vi "Process Array Elements - backup.vi"(5 "Read/Write Options":T1, 7 "Format String (%#0.15f)":string="%#0.15f", 8 "Error In":errorcluster, 9 "Name In":string, 10 "Array Variant":variant, 11 "Queue In":refnum<queue>) -> (0 "Error Out":errorcluster, 1 "Data Out":string, 3 "Queue Out":refnum<queue>)   [LabVIEW 2020]
doc: "This VI was created for use with the Read/Write Cluster VIs. It converts array elements of the cluster to strings to be written to file.\n\nFreeware from Moore Good Ideas, www.mooregoodideas.com. Do not remove this line."
uses:
  <vilib>/Utility/VariantDataType/VariantType.lvlib
  <vilib>/Utility/Data Type/NI_Data Type.lvlib
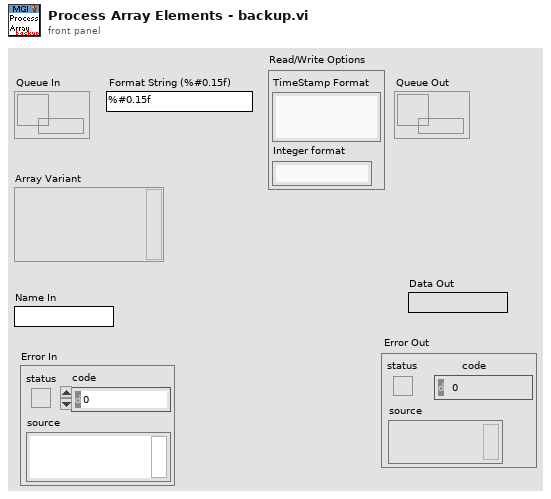
[diagram p1: front panel]
types:
  T1 = cluster{"TimeStamp Format":string, "Integer format":string}
  T2 = typedef "NI_Data Type.lvlib/Data Type.ctl" = enum8{"Invalid Type", "Void", "I8", "I16", "I32", "I64", "U8", "U16", "U32", "U64", "Single Float", "Double Float", "Extended Float", "Single Complex", "Double Complex", "Extended Complex", "Enum U8", "Enum U16", "Enum U32", "Enum U64", "Single Float With Unit", "Double Float With Unit", "Extended Float With Unit", "Single Complex with Unit", "Double Complex with Unit", "Extended Complex with Unit", "Boolean", "String", "Path", "Picture", "Tag", "Array", "Cluster", "Variant", "LV Variant", "Waveform", "Timestamp", "Digital Waveform", "Digital Data", "ExpressData", "Refnum", "External Data", "VI", "Poly VI", "LabVIEW Class Instance", "Fixed Point", "Set Collection", "Map Collection"}
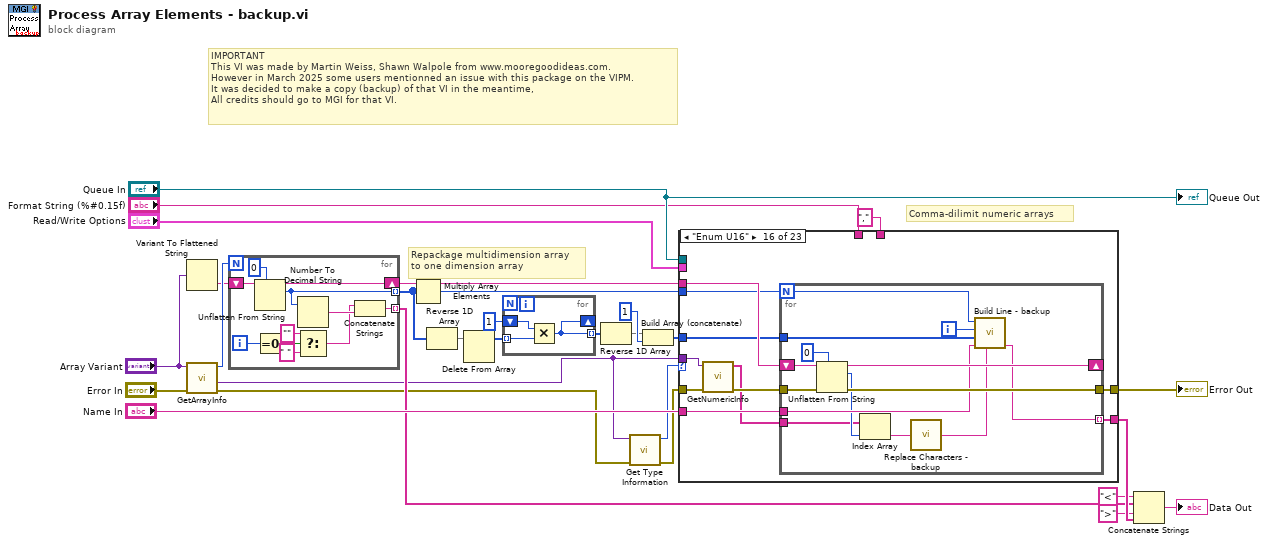
[diagram p0: block diagram]
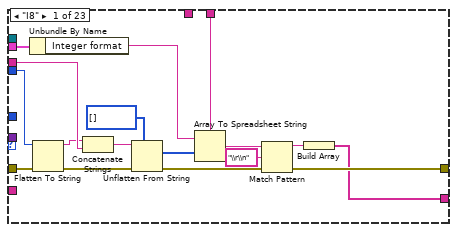
[diagram p2: hidden frame]
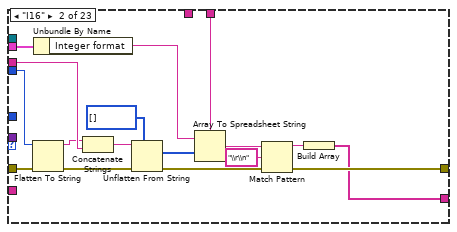
[diagram p3: hidden frame]
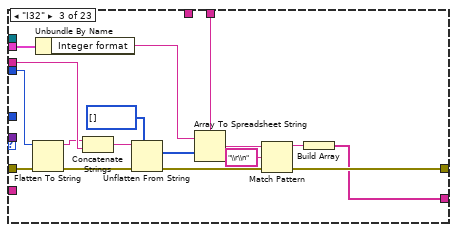
[diagram p4: hidden frame]
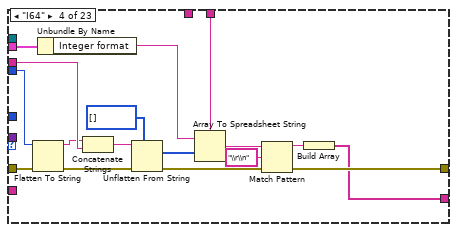
[diagram p5: hidden frame]
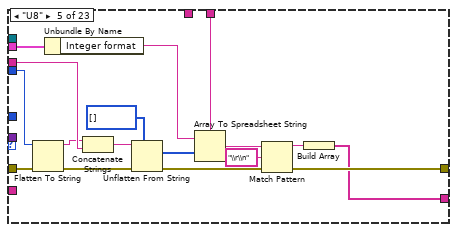
[diagram p6: hidden frame]
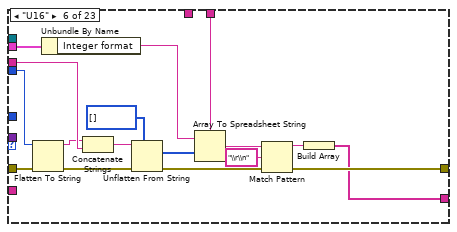
[diagram p7: hidden frame]
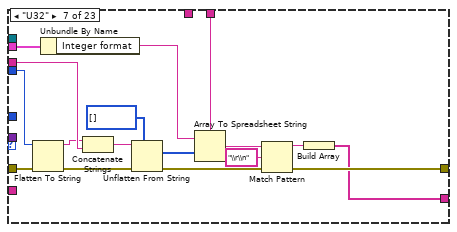
[diagram p8: hidden frame]
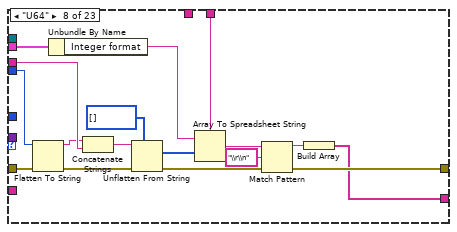
[diagram p9: hidden frame]
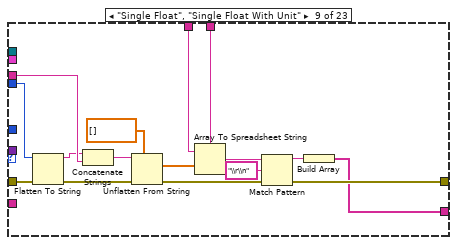
[diagram p10: hidden frame]
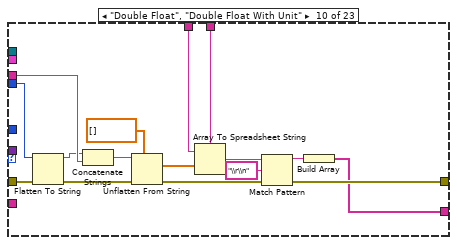
[diagram p11: hidden frame]
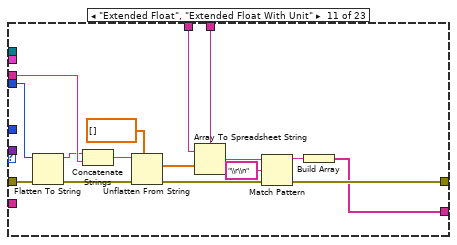
[diagram p12: hidden frame]
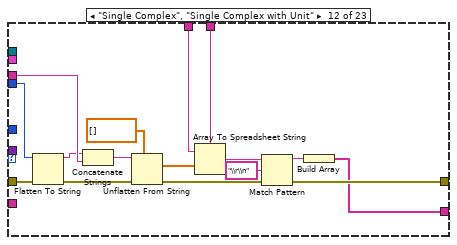
[diagram p13: hidden frame]
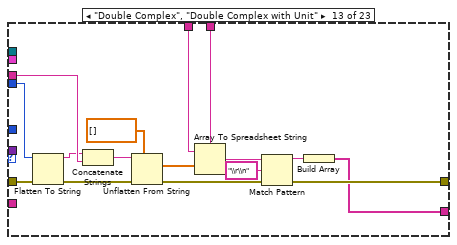
[diagram p14: hidden frame]
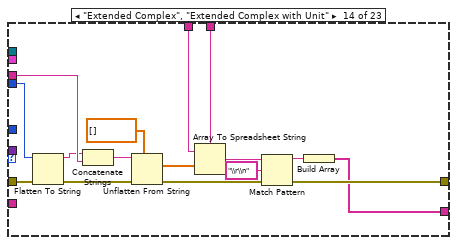
[diagram p15: hidden frame]
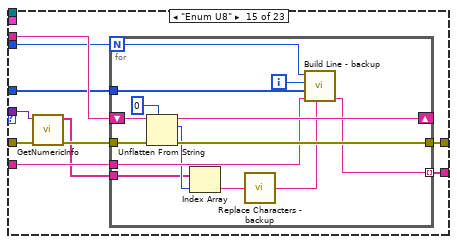
[diagram p16: hidden frame]
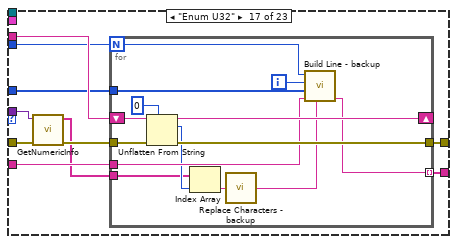
[diagram p17: hidden frame]
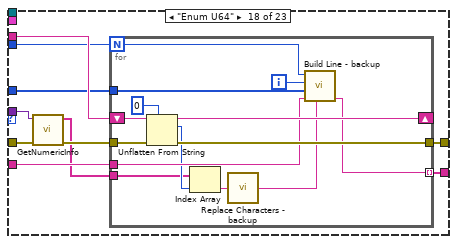
[diagram p18: hidden frame]
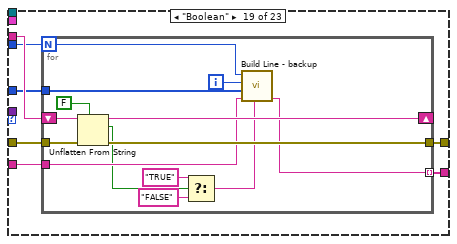
[diagram p19: hidden frame]
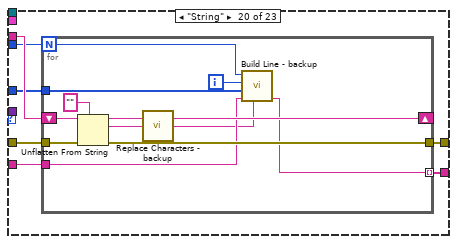
[diagram p20: hidden frame]
diagram:
  # "IMPORTANT\nThis VI was made by Martin Weiss, Shawn Walpole from www.mooregoodideas.com.\nHowever in March 2025 some users mentionned an issue with this package on the VIPM.\nIt was decided to make a copy (backup) of that VI in the meantime,\nAll credits should go to MGI for that VI."
  # "Comma-dilimit numeric arrays"
  # "Repackage multidimension array\nto one dimension array"
  n1 = Variant To Flattened String(Variant="Array Variant") -> (data string=w26:string)  [unwired: 1 out]
  n2 = call <vilib>:"GetArrayInfo.vi"("error in (no error)"="Error In", "Variant"="Array Variant") -> ("error out"=w3:errorcluster, "ArrayElement"=w4:variant, "NDims"=w27:i32)  [unwired: 6 in, 1 out]
  n3 = for {
    N: w27 -> [_]
    shift-right: [w38] -> w25
    shift-left: w26 -> [w39]
    tunnel: [w35] -> w14 mode=indexing
    tunnel: [w36] -> w10 mode=indexing
    i -> [w34]
    n4 = Unflatten From String(type=u32 0, binary string=w39) -> (rest of the binary string=w38:string, value=w35:u32)  [unwired: 3 in, 1 out]
    n5 = Equal To 0?(x=w34) -> (x = 0?=w33:bool)
    n6 = Number To Decimal String(number=w35) -> (decimal integer string=w37:string)  [unwired: 1 in]
    n7 = Select(t="", s=w33, f=" ") -> (s? t:f=w31:string)
    n8 = Concatenate Strings(w31, w37) -> (w36:string)
  }
  n9 = Multiply Array Elements(1:w14) -> (0:w24:u32)
  n10 = Reverse 1D Array(array=w14) -> (reversed array=w15:u32[])
  n11 = Delete From Array(array=w15) -> (array with subset deleted=w16:u32[])  [unwired: 2 in, 1 out]
  n12 = for {
    tunnel: w16 -> [w43] mode=indexing
    shift-right: [w41] -> _
    shift-left: i8 1 -> [w42]
    tunnel: [w41] -> w18 mode=indexing
    n13 = Multiply(x=w42, y=w43) -> (x*y=w41:u32)
  }
  n14 = Reverse 1D Array(array=w18) -> (reversed array=w19:u32[])
  n15 = call <vilib>:"Get Type Information.vi"("error in (no error)"=w3, "variant"=w4) -> ("error out"=w1:errorcluster, "type"=w2:T2)  [unwired: 5 in, 3 out]
  n16 = Build Array (concatenate)(w19, i8 1) -> (w13:u32[])
  n17 = case shown="\"Enum U16\"" w2 {
    tunnel: [w59 w75 w91 w107 w123 w139 w155 w171 w186 w201 w216 w231 w246 w261 w271 w295 w319 w343 w364 w385 w404 w420 w430] -> w12
    tunnel: w1 -> [w48 w64 w80 w96 w112 w128 w144 w160 w175 w190 w205 w220 w235 w250 w264 w288 w312 w336 w363 w384 w403 w420 w438]
    tunnel: w25 -> [w58 w74 w90 w106 w122 w138 w154 w170 w185 w200 w215 w230 w245 w260 w270 w294 w318 w342 w362 w383 w402 w419 w425]
    tunnel: w24 -> [w57 w73 w89 w105 w121 w137 w153 w169 w184 w199 w214 w229 w244 w259 w269 w293 w317 w341 w361 w382 w401 _ w437]
    tunnel: "Name In" -> [_ _ _ _ _ _ _ _ _ _ _ _ _ _ w268 w292 w316 w340 w360 w381 w400 _ w436]
    tunnel: [w56 w72 w88 w104 w120 w136 w152 w168 w183 w198 w213 w228 w243 w258 w266 w290 w314 w338 w358 w379 w398 w418 _] -> w22
    tunnel: w13 -> [_ _ _ _ _ _ _ _ _ _ _ _ _ _ w267 w291 w315 w339 w359 w380 w399 _ w435]
    tunnel: "Queue In" -> [_ _ _ _ _ _ _ _ _ _ _ _ _ _ _ _ _ _ _ _ _ _ w431]
    tunnel: w4 -> [_ _ _ _ _ _ _ _ _ _ _ _ _ _ w265 w289 w313 w337 _ _ _ _ w428]
    tunnel: "Format String (%#0.15f)" -> [_ _ _ _ _ _ _ _ w173 w188 w203 w218 w233 w248 _ _ _ _ _ _ _ _ _]
    tunnel: "," ("delimiter (Tab)") -> [w46 w62 w78 w94 w110 w126 w142 w158 w172 w187 w202 w217 w232 w247 _ _ _ _ _ _ _ _ _]
    tunnel: "Read/Write Options" -> [w45 w61 w77 w93 w109 w125 w141 w157 _ _ _ _ _ _ _ _ _ _ _ _ _ _ _]
    frame "I8" {
      n18 = Unbundle By Name(w45) -> ("Integer format"=w44:string)
      n19 = Flatten To String(anything=w57, error in (no error)=w48) -> (data string=w53:string, error out=w47:errorcluster)  [unwired: 2 in, 1 out]
      n20 = Concatenate Strings(w53, w58) -> (w54:string)
      n21 = Unflatten From String(type=i8[] [], binary string=w54, error in (no error)=w47) -> (value=w50:i8[], error out=w59:errorcluster)  [unwired: 2 in, 1 out]
      n22 = Array To Spreadsheet String(delimiter (Tab)=w46, array=w50, 3:w44) -> (spreadsheet string=w52:string)
      n23 = Match Pattern(string=w52, regular expression="\\r\\n") -> (before substring=w49:string)  [unwired: 1 in, 3 out]
      n24 = Build Array(w49) -> (w56:string[])
    }
    frame "I16" {
      n25 = Flatten To String(anything=w73, error in (no error)=w64) -> (data string=w69:string, error out=w63:errorcluster)  [unwired: 2 in, 1 out]
      n26 = Unbundle By Name(w61) -> ("Integer format"=w60:string)
      n27 = Concatenate Strings(w69, w74) -> (w70:string)
      n28 = Unflatten From String(type=i16[] [], binary string=w70, error in (no error)=w63) -> (value=w66:i16[], error out=w75:errorcluster)  [unwired: 2 in, 1 out]
      n29 = Array To Spreadsheet String(delimiter (Tab)=w62, array=w66, 3:w60) -> (spreadsheet string=w68:string)
      n30 = Match Pattern(string=w68, regular expression="\\r\\n") -> (before substring=w65:string)  [unwired: 1 in, 3 out]
      n31 = Build Array(w65) -> (w72:string[])
    }
    frame "I32" {
      n32 = Flatten To String(anything=w89, error in (no error)=w80) -> (data string=w85:string, error out=w79:errorcluster)  [unwired: 2 in, 1 out]
      n33 = Unbundle By Name(w77) -> ("Integer format"=w76:string)
      n34 = Concatenate Strings(w85, w90) -> (w86:string)
      n35 = Unflatten From String(type=i32[] [], binary string=w86, error in (no error)=w79) -> (value=w82:i32[], error out=w91:errorcluster)  [unwired: 2 in, 1 out]
      n36 = Array To Spreadsheet String(delimiter (Tab)=w78, array=w82, 3:w76) -> (spreadsheet string=w84:string)
      n37 = Match Pattern(string=w84, regular expression="\\r\\n") -> (before substring=w81:string)  [unwired: 1 in, 3 out]
      n38 = Build Array(w81) -> (w88:string[])
    }
    frame "I64" {
      n39 = Flatten To String(anything=w105, error in (no error)=w96) -> (data string=w101:string, error out=w95:errorcluster)  [unwired: 2 in, 1 out]
      n40 = Unbundle By Name(w93) -> ("Integer format"=w92:string)
      n41 = Concatenate Strings(w101, w106) -> (w102:string)
      n42 = Unflatten From String(type=i64[] [], binary string=w102, error in (no error)=w95) -> (value=w98:i64[], error out=w107:errorcluster)  [unwired: 2 in, 1 out]
      n43 = Array To Spreadsheet String(delimiter (Tab)=w94, array=w98, 3:w92) -> (spreadsheet string=w100:string)
      n44 = Match Pattern(string=w100, regular expression="\\r\\n") -> (before substring=w97:string)  [unwired: 1 in, 3 out]
      n45 = Build Array(w97) -> (w104:string[])
    }
    frame "U8" {
      n46 = Flatten To String(anything=w121, error in (no error)=w112) -> (data string=w117:string, error out=w111:errorcluster)  [unwired: 2 in, 1 out]
      n47 = Unbundle By Name(w109) -> ("Integer format"=w108:string)
      n48 = Concatenate Strings(w117, w122) -> (w118:string)
      n49 = Unflatten From String(type=u8[] [], binary string=w118, error in (no error)=w111) -> (value=w114:u8[], error out=w123:errorcluster)  [unwired: 2 in, 1 out]
      n50 = Array To Spreadsheet String(delimiter (Tab)=w110, array=w114, 3:w108) -> (spreadsheet string=w116:string)
      n51 = Match Pattern(string=w116, regular expression="\\r\\n") -> (before substring=w113:string)  [unwired: 1 in, 3 out]
      n52 = Build Array(w113) -> (w120:string[])
    }
    frame "U16" {
      n53 = Flatten To String(anything=w137, error in (no error)=w128) -> (data string=w133:string, error out=w127:errorcluster)  [unwired: 2 in, 1 out]
      n54 = Unbundle By Name(w125) -> ("Integer format"=w124:string)
      n55 = Concatenate Strings(w133, w138) -> (w134:string)
      n56 = Unflatten From String(type=u16[] [], binary string=w134, error in (no error)=w127) -> (value=w130:u16[], error out=w139:errorcluster)  [unwired: 2 in, 1 out]
      n57 = Array To Spreadsheet String(delimiter (Tab)=w126, array=w130, 3:w124) -> (spreadsheet string=w132:string)
      n58 = Match Pattern(string=w132, regular expression="\\r\\n") -> (before substring=w129:string)  [unwired: 1 in, 3 out]
      n59 = Build Array(w129) -> (w136:string[])
    }
    frame "U32" {
      n60 = Flatten To String(anything=w153, error in (no error)=w144) -> (data string=w149:string, error out=w143:errorcluster)  [unwired: 2 in, 1 out]
      n61 = Unbundle By Name(w141) -> ("Integer format"=w140:string)
      n62 = Concatenate Strings(w149, w154) -> (w150:string)
      n63 = Unflatten From String(type=u32[] [], binary string=w150, error in (no error)=w143) -> (value=w146:u32[], error out=w155:errorcluster)  [unwired: 2 in, 1 out]
      n64 = Array To Spreadsheet String(delimiter (Tab)=w142, array=w146, 3:w140) -> (spreadsheet string=w148:string)
      n65 = Match Pattern(string=w148, regular expression="\\r\\n") -> (before substring=w145:string)  [unwired: 1 in, 3 out]
      n66 = Build Array(w145) -> (w152:string[])
    }
    frame "U64" {
      n67 = Flatten To String(anything=w169, error in (no error)=w160) -> (data string=w165:string, error out=w159:errorcluster)  [unwired: 2 in, 1 out]
      n68 = Unbundle By Name(w157) -> ("Integer format"=w156:string)
      n69 = Concatenate Strings(w165, w170) -> (w166:string)
      n70 = Unflatten From String(type=u64[] [], binary string=w166, error in (no error)=w159) -> (value=w162:u64[], error out=w171:errorcluster)  [unwired: 2 in, 1 out]
      n71 = Array To Spreadsheet String(delimiter (Tab)=w158, array=w162, 3:w156) -> (spreadsheet string=w164:string)
      n72 = Match Pattern(string=w164, regular expression="\\r\\n") -> (before substring=w161:string)  [unwired: 1 in, 3 out]
      n73 = Build Array(w161) -> (w168:string[])
    }
    frame "Single Float", "Single Float With Unit" {
      n74 = Flatten To String(anything=w184, error in (no error)=w175) -> (data string=w180:string, error out=w174:errorcluster)  [unwired: 2 in, 1 out]
      n75 = Concatenate Strings(w180, w185) -> (w181:string)
      n76 = Unflatten From String(type=sgl[] [], binary string=w181, error in (no error)=w174) -> (value=w177:sgl[], error out=w186:errorcluster)  [unwired: 2 in, 1 out]
      n77 = Array To Spreadsheet String(delimiter (Tab)=w172, array=w177, 3:w173) -> (spreadsheet string=w179:string)
      n78 = Match Pattern(string=w179, regular expression="\\r\\n") -> (before substring=w176:string)  [unwired: 1 in, 3 out]
      n79 = Build Array(w176) -> (w183:string[])
    }
    frame "Double Float", "Double Float With Unit" {
      n80 = Flatten To String(anything=w199, error in (no error)=w190) -> (data string=w195:string, error out=w189:errorcluster)  [unwired: 2 in, 1 out]
      n81 = Concatenate Strings(w195, w200) -> (w196:string)
      n82 = Unflatten From String(type=dbl[] [], binary string=w196, error in (no error)=w189) -> (value=w192:dbl[], error out=w201:errorcluster)  [unwired: 2 in, 1 out]
      n83 = Array To Spreadsheet String(delimiter (Tab)=w187, array=w192, 3:w188) -> (spreadsheet string=w194:string)
      n84 = Match Pattern(string=w194, regular expression="\\r\\n") -> (before substring=w191:string)  [unwired: 1 in, 3 out]
      n85 = Build Array(w191) -> (w198:string[])
    }
    frame "Extended Float", "Extended Float With Unit" {
      n86 = Flatten To String(anything=w214, error in (no error)=w205) -> (data string=w210:string, error out=w204:errorcluster)  [unwired: 2 in, 1 out]
      n87 = Concatenate Strings(w210, w215) -> (w211:string)
      n88 = Unflatten From String(type=ext[] [], binary string=w211, error in (no error)=w204) -> (value=w207:ext[], error out=w216:errorcluster)  [unwired: 2 in, 1 out]
      n89 = Array To Spreadsheet String(delimiter (Tab)=w202, array=w207, 3:w203) -> (spreadsheet string=w209:string)
      n90 = Match Pattern(string=w209, regular expression="\\r\\n") -> (before substring=w206:string)  [unwired: 1 in, 3 out]
      n91 = Build Array(w206) -> (w213:string[])
    }
    frame "Single Complex", "Single Complex with Unit" {
      n92 = Flatten To String(anything=w229, error in (no error)=w220) -> (data string=w225:string, error out=w219:errorcluster)  [unwired: 2 in, 1 out]
      n93 = Concatenate Strings(w225, w230) -> (w226:string)
      n94 = Unflatten From String(type=csg[] [], binary string=w226, error in (no error)=w219) -> (value=w222:csg[], error out=w231:errorcluster)  [unwired: 2 in, 1 out]
      n95 = Array To Spreadsheet String(delimiter (Tab)=w217, array=w222, 3:w218) -> (spreadsheet string=w224:string)
      n96 = Match Pattern(string=w224, regular expression="\\r\\n") -> (before substring=w221:string)  [unwired: 1 in, 3 out]
      n97 = Build Array(w221) -> (w228:string[])
    }
    frame "Double Complex", "Double Complex with Unit" {
      n98 = Flatten To String(anything=w244, error in (no error)=w235) -> (data string=w240:string, error out=w234:errorcluster)  [unwired: 2 in, 1 out]
      n99 = Concatenate Strings(w240, w245) -> (w241:string)
      n100 = Unflatten From String(type=cdb[] [], binary string=w241, error in (no error)=w234) -> (value=w237:cdb[], error out=w246:errorcluster)  [unwired: 2 in, 1 out]
      n101 = Array To Spreadsheet String(delimiter (Tab)=w232, array=w237, 3:w233) -> (spreadsheet string=w239:string)
      n102 = Match Pattern(string=w239, regular expression="\\r\\n") -> (before substring=w236:string)  [unwired: 1 in, 3 out]
      n103 = Build Array(w236) -> (w243:string[])
    }
    frame "Extended Complex", "Extended Complex with Unit" {
      n104 = Flatten To String(anything=w259, error in (no error)=w250) -> (data string=w255:string, error out=w249:errorcluster)  [unwired: 2 in, 1 out]
      n105 = Concatenate Strings(w255, w260) -> (w256:string)
      n106 = Unflatten From String(type=cxt[] [], binary string=w256, error in (no error)=w249) -> (value=w252:cxt[], error out=w261:errorcluster)  [unwired: 2 in, 1 out]
      n107 = Array To Spreadsheet String(delimiter (Tab)=w247, array=w252, 3:w248) -> (spreadsheet string=w254:string)
      n108 = Match Pattern(string=w254, regular expression="\\r\\n") -> (before substring=w251:string)  [unwired: 1 in, 3 out]
      n109 = Build Array(w251) -> (w258:string[])
    }
    frame "Enum U8" {
      n110 = call <vilib>:"GetNumericInfo.vi"("error in (no error)"=w264, "Variant"=w265) -> ("error out"=w263:errorcluster, "EnumNames"=w262:string[])  [unwired: 6 in, 2 out]
      n111 = for {
        N: w269 -> [w281]
        tunnel: [w282] -> w271
        tunnel: w263 -> [w283]
        shift-right: [w284] -> _
        shift-left: w270 -> [w285]
        tunnel: w268 -> [w277]
        tunnel: [w278] -> w266 mode=indexing
        tunnel: w267 -> [w279]
        tunnel: w262 -> [w274]
        i -> [w280]
        n112 = Unflatten From String(type=u8 0, binary string=w285, error in (no error)=w283) -> (rest of the binary string=w284:string, value=w275:u8, error out=w282:errorcluster)  [unwired: 2 in]
        n113 = Index Array(array=w274, index=w275) -> (element=w273:string)
        n114 = call "Replace Characters - backup.vi"("String In"=w273) -> ("String Out"=w272:string)  [unwired: 1 in]
        n115 = call "Build Line - backup.vi"("Value String (\"\")"=w272, "Name In"=w277, "Array"=w279, "Iteration"=w280, "Iterations"=w281) -> ("Line"=w278:string)  [unwired: 5 in, 1 out]
      }
    }
    frame "Enum U16" {
      n116 = call <vilib>:"GetNumericInfo.vi"("error in (no error)"=w288, "Variant"=w289) -> ("error out"=w287:errorcluster, "EnumNames"=w286:string[])  [unwired: 6 in, 2 out]
      n117 = for {
        N: w293 -> [w305]
        tunnel: [w306] -> w295
        tunnel: w287 -> [w307]
        shift-right: [w308] -> _
        shift-left: w294 -> [w309]
        tunnel: w292 -> [w301]
        tunnel: [w302] -> w290 mode=indexing
        tunnel: w291 -> [w303]
        tunnel: w286 -> [w298]
        i -> [w304]
        n118 = Unflatten From String(type=u16 0, binary string=w309, error in (no error)=w307) -> (rest of the binary string=w308:string, value=w299:u16, error out=w306:errorcluster)  [unwired: 2 in]
        n119 = Index Array(array=w298, index=w299) -> (element=w297:string)
        n120 = call "Replace Characters - backup.vi"("String In"=w297) -> ("String Out"=w296:string)  [unwired: 1 in]
        n121 = call "Build Line - backup.vi"("Value String (\"\")"=w296, "Name In"=w301, "Array"=w303, "Iteration"=w304, "Iterations"=w305) -> ("Line"=w302:string)  [unwired: 5 in, 1 out]
      }
    }
    frame "Enum U32" {
      n122 = call <vilib>:"GetNumericInfo.vi"("error in (no error)"=w312, "Variant"=w313) -> ("error out"=w311:errorcluster, "EnumNames"=w310:string[])  [unwired: 6 in, 2 out]
      n123 = for {
        N: w317 -> [w329]
        tunnel: [w330] -> w319
        tunnel: w311 -> [w331]
        shift-right: [w332] -> _
        shift-left: w318 -> [w333]
        tunnel: w316 -> [w325]
        tunnel: [w326] -> w314 mode=indexing
        tunnel: w315 -> [w327]
        tunnel: w310 -> [w322]
        i -> [w328]
        n124 = Unflatten From String(type=u32 0, binary string=w333, error in (no error)=w331) -> (rest of the binary string=w332:string, value=w323:u32, error out=w330:errorcluster)  [unwired: 2 in]
        n125 = Index Array(array=w322, index=w323) -> (element=w321:string)
        n126 = call "Replace Characters - backup.vi"("String In"=w321) -> ("String Out"=w320:string)  [unwired: 1 in]
        n127 = call "Build Line - backup.vi"("Value String (\"\")"=w320, "Name In"=w325, "Array"=w327, "Iteration"=w328, "Iterations"=w329) -> ("Line"=w326:string)  [unwired: 5 in, 1 out]
      }
    }
    frame "Enum U64" {
      n128 = call <vilib>:"GetNumericInfo.vi"("error in (no error)"=w336, "Variant"=w337) -> ("error out"=w335:errorcluster, "EnumNames"=w334:string[])  [unwired: 6 in, 2 out]
      n129 = for {
        N: w341 -> [w353]
        tunnel: [w354] -> w343
        tunnel: w335 -> [w355]
        shift-right: [w356] -> _
        shift-left: w342 -> [w357]
        tunnel: w340 -> [w349]
        tunnel: [w350] -> w338 mode=indexing
        tunnel: w339 -> [w351]
        tunnel: w334 -> [w346]
        i -> [w352]
        n130 = Unflatten From String(type=u64 0, binary string=w357, error in (no error)=w355) -> (rest of the binary string=w356:string, value=w347:u64, error out=w354:errorcluster)  [unwired: 2 in]
        n131 = Index Array(array=w346, index=w347) -> (element=w345:string)
        n132 = call "Replace Characters - backup.vi"("String In"=w345) -> ("String Out"=w344:string)  [unwired: 1 in]
        n133 = call "Build Line - backup.vi"("Value String (\"\")"=w344, "Name In"=w349, "Array"=w351, "Iteration"=w352, "Iterations"=w353) -> ("Line"=w350:string)  [unwired: 5 in, 1 out]
      }
    }
    frame "Boolean" {
      n134 = for {
        N: w361 -> [w374]
        tunnel: [w375] -> w364
        tunnel: w363 -> [w376]
        shift-right: [w377] -> _
        shift-left: w362 -> [w378]
        tunnel: w360 -> [w370]
        tunnel: [w371] -> w358 mode=indexing
        tunnel: w359 -> [w372]
        i -> [w373]
        n135 = Unflatten From String(type=FALSE, binary string=w378, error in (no error)=w376) -> (rest of the binary string=w377:string, value=w366:bool, error out=w375:errorcluster)  [unwired: 2 in]
        n136 = Select(t="TRUE", s=w366, f="FALSE") -> (s? t:f=w365:string)
        n137 = call "Build Line - backup.vi"("Value String (\"\")"=w365, "Name In"=w370, "Array"=w372, "Iteration"=w373, "Iterations"=w374) -> ("Line"=w371:string)  [unwired: 5 in, 1 out]
      }
    }
    frame "String" {
      n138 = for {
        N: w382 -> [w393]
        tunnel: [w394] -> w385
        tunnel: w384 -> [w395]
        shift-right: [w396] -> _
        shift-left: w383 -> [w397]
        tunnel: w381 -> [w389]
        tunnel: [w390] -> w379 mode=indexing
        tunnel: w380 -> [w391]
        i -> [w392]
        n139 = Unflatten From String(type="", binary string=w397, error in (no error)=w395) -> (rest of the binary string=w396:string, value=w387:string, error out=w394:errorcluster)  [unwired: 2 in]
        n140 = call "Replace Characters - backup.vi"("String In"=w387) -> ("String Out"=w386:string)  [unwired: 1 in]
        n141 = call "Build Line - backup.vi"("Value String (\"\")"=w386, "Name In"=w389, "Array"=w391, "Iteration"=w392, "Iterations"=w393) -> ("Line"=w390:string)  [unwired: 5 in, 1 out]
      }
    }
    frame "Path" {
      n142 = for {
        N: w401 -> [w413]
        tunnel: [w414] -> w404
        tunnel: w403 -> [w415]
        shift-right: [w416] -> _
        shift-left: w402 -> [w417]
        tunnel: w400 -> [w409]
        tunnel: [w410] -> w398 mode=indexing
        tunnel: w399 -> [w411]
        i -> [w412]
        n143 = Unflatten From String(type=path "", binary string=w417, error in (no error)=w415) -> (rest of the binary string=w416:string, value=w407:path, error out=w414:errorcluster)  [unwired: 2 in]
        n144 = Path To String(path=w407) -> (string=w406:string)
        n145 = call "Replace Characters - backup.vi"("String In"=w406) -> ("String Out"=w405:string)  [unwired: 1 in]
        n146 = call "Build Line - backup.vi"("Value String (\"\")"=w405, "Name In"=w409, "Array"=w411, "Iteration"=w412, "Iterations"=w413) -> ("Line"=w410:string)  [unwired: 5 in, 1 out]
      }
    }
    frame Default {
      n147 = String To Byte Array(string=w419) -> (unsigned byte array=w424:u8[])
      n148 = Number To Hexadecimal String(1:i16 2 ("width (-)"), 2:w424) -> (0:w423:string[])
      n149 = Build Array (concatenate)("0x", w423) -> (w418:string[])
    }
    frame "Cluster" {
      # "Enqueue cluster\nelements"
      n150 = Variant To Flattened String(Variant=w428) -> (1:w427:i16[])  [unwired: 1 out]
      n151 = for {
        N: w437 -> [w457]
        tunnel: [w451] -> w432
        tunnel: w438 -> [w453]
        tunnel: w436 -> [w448]
        tunnel: w435 -> [w455]
        tunnel: [w449] -> w433 mode=indexing
        tunnel: [w454] -> w429 mode=indexing
        tunnel: w427 -> [w452]
        shift-right: [w445] -> _
        shift-left: w425 -> [w446]
        i -> [w456]
        n152 = Flattened String To Variant(4:w453, 6:w446, 7:w452) -> (0:w451:errorcluster, 3:w449:variant)
        n153 = Variant To Flattened String(Variant=w449) -> (data string=w450:string)  [unwired: 1 out]
        n154 = String Length(string=w450) -> (length=w447:i32)
        n155 = String Subset(string=w446, offset (0)=w447) -> (substring=w445:string)  [unwired: 1 in]
        n156 = call "Build Line - backup.vi"("Name In"=w448, "Array"=w455, "Iteration"=w456, "Iterations"=w457) -> ("Name Out"=w454:string)  [unwired: 6 in, 1 out]
      }
      n157 = Reverse 1D Array(array=w429) -> (reversed array=w426:string[])
      n158 = Reverse 1D Array(array=w433) -> (reversed array=w434:variant[])
      n159 = for {
        tunnel: [w444] -> w430
        tunnel: w434 -> [w443] mode=indexing
        tunnel: w432 -> [w442]
        tunnel: w431 -> [w440]
        tunnel: w426 -> [w439] mode=indexing
        n160 = Bundle("Variant"=w443, "Name Out"=w439) -> (w441:cluster{"Variant":variant, "Name Out":string})  [unwired: 1 in]
        n161 = Enqueue Element At Opposite End(queue=w440, element=w441, error in (no error)=w442) -> (error out=w444:errorcluster)  [unwired: 1 in, 2 out]
      }
    }
  }
  "Error Out" <- w12
  n162 = Concatenate Strings("<", w10, ">", w22) -> (→"Data Out":string)
  "Queue Out" <- "Queue In"
